vi "Draw.vi"(8 "error in (no error)":errorcluster, 10 "Picture in":picture, 11 "Graphic In":refnum<class "Graphic.lvclass">) -> (0 "error out":errorcluster, 2 "Picture out":picture, 3 "Graphic Out":refnum<class "Graphic.lvclass">)   [LabVIEW 2017, in "Graphic.lvclass"]
doc: "Draw the graphic into the picture."
uses:
  Graphic.lvclass
  Graphic.lvclass/Graphic.ctl
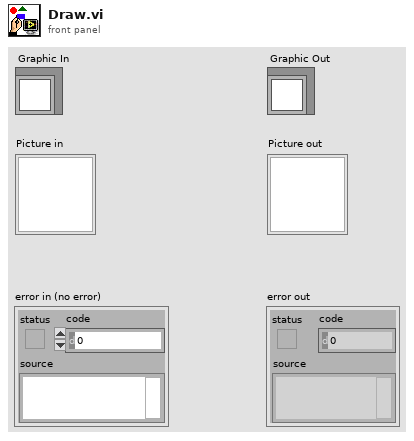
[diagram p1: front panel]
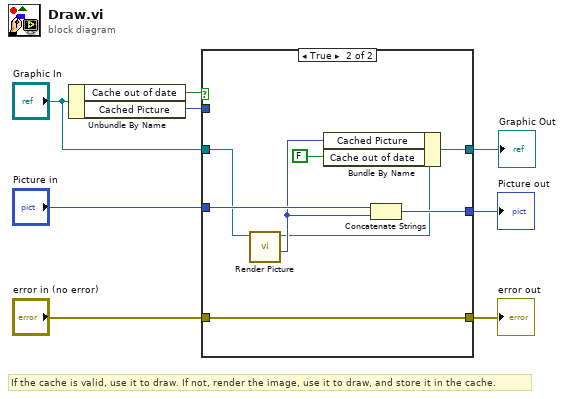
[diagram p0: block diagram]
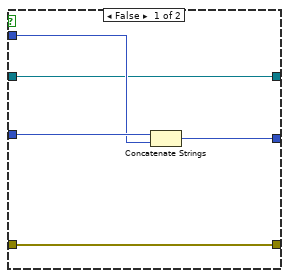
[diagram p2: hidden frame]
diagram:
  # "If the cache is valid, use it to draw. If not, render the image, use it to draw, and store it in the cache."
  n1 = Unbundle By Name("Graphic In") -> ("Cache out of date"=w8:bool, "Cached Picture"=w7:picture)
  n2 = case shown="True" w8 {
    tunnel: w7 -> [w11 _]
    tunnel: [w10 w20] -> w6
    tunnel: "Graphic In" -> [w9 w19]
    tunnel: [w13 w14] -> w4
    tunnel: "error in (no error)" -> [w13 w14]
    tunnel: "Picture in" -> [w12 w21]
    tunnel: [w9 w16] -> w1
    frame False {
      n3 = Concatenate Strings(w12, w11) -> (w10:picture)
    }
    frame True {
      n4 = call-dynamic "Render Picture.vi"("Graphic In"=w19) -> ("Picture"=w18:picture, "Graphic Out"=w15:refnum<class "Graphic.lvclass">)  [unwired: 9 out]
      n5 = Bundle By Name(cluster=w15, "Cached Picture"=w18, "Cache out of date"=FALSE) -> (w16:refnum<class "Graphic.lvclass">)
      n6 = Concatenate Strings(w21, w18) -> (w20:picture)
    }
  }
  "Picture out" <- w6
  "Graphic Out" <- w1
  "error out" <- w4
